vi "Get_Status.vi"(5 "Device Number":T1, 7 "Update":bool) -> (2 "Status":T4 {"OP Status" items=["INITIALIZING", "SELFTEST_IN_PROGRESS", "ERROR", "IMU_AUTOCAL_IN_PROGRESS", "NORMAL"]; "Calibration Status" items=["IMU_CAL_STATE_MASK"=3, "IMU_CAL_STATE_INPROGRESS"=0, "IMU_CAL_STATE_ACCUMULATE"=1, "IMU_CAL_STATE_COMPLETE"=2]})   [LabVIEW 2019]
doc: "This navX VI returns the current status of the navX."
uses:
  _TypeDefs/Flags/Z900_navX_Flags_OpStatusTypeDef.ctl
  _TypeDefs/Flags/Z900_navX_Flags_CalibrationStatusTypeDef.ctl
  _TypeDefs/FRIC_navX_DeviceNumbersTypeDef.ctl
  _TypeDefs/Z900_navX_DeviceRegisters.ctl
  _TypeDefs/Flags/Z900_navX_Flags_SelfTestStatusTypeDef.ctl
  _Util/Z900_navX_Util_LittleEndian_to_BigEndian.vi
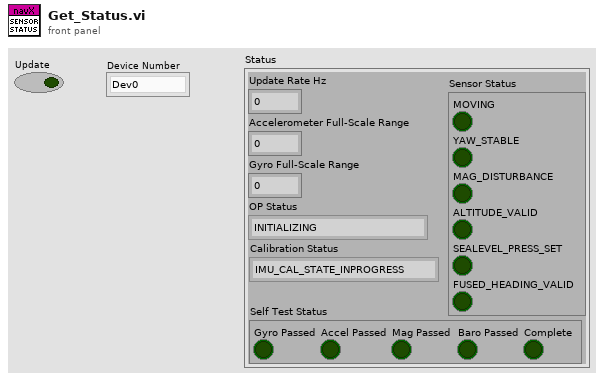
[diagram p1: front panel]
types:
  T1 = typedef "FRIC_navX_DeviceNumbersTypeDef.ctl" = enum16{"Dev0", "Dev1", "Dev2", "Dev3"}
  T2 = typedef "Z900_navX_Flags_OpStatusTypeDef.ctl" = u8
  T3 = typedef "Z900_navX_Flags_CalibrationStatusTypeDef.ctl" = u8
  T4 = cluster{"Update Rate Hz":u8, "Accelerometer Full-Scale Range":u8, "Gyro Full-Scale Range":u16, "OP Status":T2, "Calibration Status":T3, "Sensor Status":cluster{"MOVING":bool, "YAW_STABLE":bool, "MAG_DISTURBANCE":bool, "ALTITUDE_VALID":bool, "SEALEVEL_PRESS_SET":bool, "FUSED_HEADING_VALID":bool}, "Self Test Status":cluster{"Gyro Passed":bool, "Accel Passed":bool, "Mag Passed":bool, "Baro Passed":bool, "Complete":bool}}
  T5 = cluster{"MOVING":bool, "YAW_STABLE":bool, "MAG_DISTURBANCE":bool, "ALTITUDE_VALID":bool, "SEALEVEL_PRESS_SET":bool, "FUSED_HEADING_VALID":bool}
  T6 = cluster{"Gyro Passed":bool, "Accel Passed":bool, "Mag Passed":bool, "Baro Passed":bool, "Complete":bool}
  T7 = typedef "Z900_navX_Flags_SelfTestStatusTypeDef.ctl" = u8
  T8 = typedef "Z900_navX_DeviceRegisters.ctl" = u8
  T9 = cluster{"Update Rate Hz":u8, "Accelerometer Full-Scale Range":u8, "Gyro Full-Scale Range":u16, "OP Status":T2, "Calibration Status":T3, "Sensor Status":cluster{"MOVING":bool, "YAW_STABLE":bool, "MAG_DISTURBANCE":bool, "ALTITUDE_VALID":bool, "SEALEVEL_PRESS_SET":bool, "FUSED_HEADING_VALID":bool}, "Self Test Status":cluster{"Gyro Passed":bool, "Accel Passed":bool, "Mag Passed":bool, "Baro Passed":bool, "Complete":bool}}[]
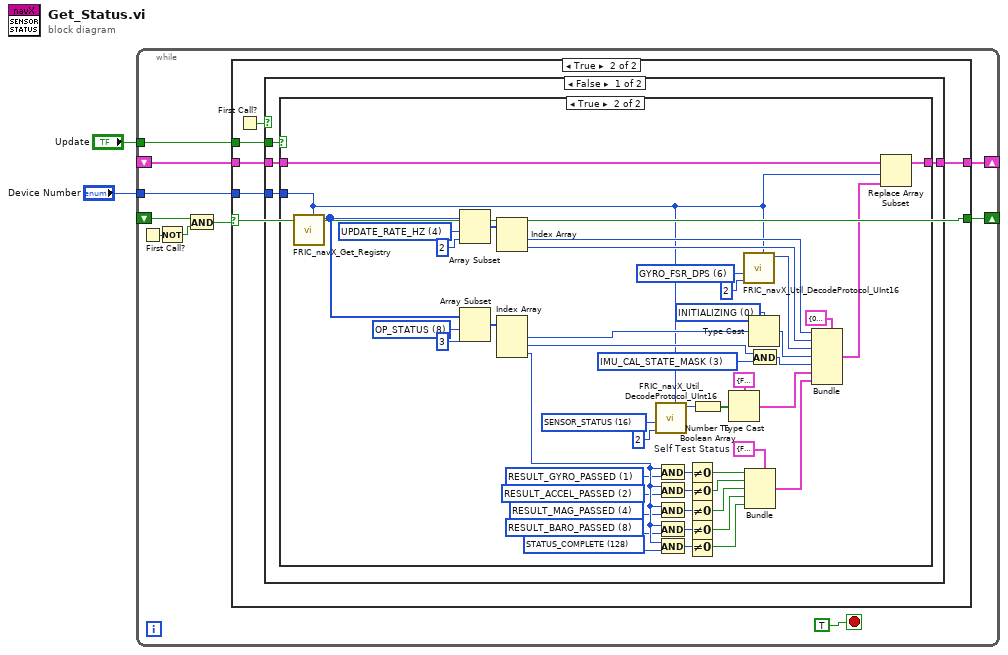
[diagram p0: block diagram]
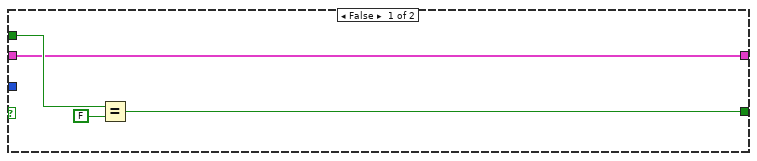
[diagram p2: hidden frame]
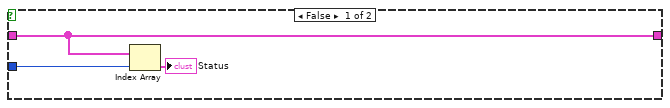
[diagram p3: hidden frame]
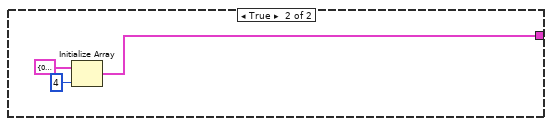
[diagram p4: hidden frame]
diagram:
  n1 = while {
    shift-right: [w12] -> _
    shift-left: _ -> [w9]
    tunnel: "Update" -> [w10]
    tunnel: "Device Number" -> [w8]
    shift-right: [w3] -> _
    shift-left: _ -> [w5]
    stop <- TRUE stop-if-true
    n2 = First Call?() -> (First Call?: T/F=w7:bool)
    n3 = Not(x=w7) -> (.not. x?=w6:bool)
    n4 = And(x=w5, y=w6) -> (x .and. y?=w4:bool)
    n5 = case shown="True" w4 {
      selector: w4 -> [_ w17]
      tunnel: [w13 w22] -> w12
      tunnel: w10 -> [w15 w21]
      tunnel: w9 -> [w13 w20]
      tunnel: w8 -> [_ w19]
      tunnel: [w14 w17] -> w3
      frame False {
        n6 = Equal?(x=w15, y=FALSE) -> (x = y?=w14:bool)
      }
      frame True {
        n7 = First Call?() -> (First Call?: T/F=w18:bool)
        n8 = case shown="False" w18 {
          tunnel: [w26 w77] -> w22
          tunnel: w21 -> [w25 _]
          tunnel: w20 -> [w24 _]
          tunnel: w19 -> [w23 _]
          frame False {
            n9 = case shown="True" w25 {
              tunnel: [w28 w32] -> w26
              tunnel: w24 -> [w28 w33]
              tunnel: w23 -> [w27 w30]
              frame False {
                n10 = Index Array(array=w28, index=w27) -> (element=→"Status":T4)
              }
              frame True {
                w34 = T6 {"Gyro Passed"=FALSE, "Accel Passed"=FALSE, "Mag Passed"=FALSE, "Baro Passed"=FALSE, "Complete"=FALSE}  # Self Test Status
                w41 = T7 128 items=["STATUS_COMPLETE"=128, "RESULT_GYRO_PASSED"=1, "RESULT_ACCEL_PASSED"=2, "RESULT_MAG_PASSED"=4, "RESULT_BARO_PASSED"=8] ("Self Test Status")
                w42 = T7 8 items=["STATUS_COMPLETE"=128, "RESULT_GYRO_PASSED"=1, "RESULT_ACCEL_PASSED"=2, "RESULT_MAG_PASSED"=4, "RESULT_BARO_PASSED"=8] ("Self Test Status")
                w45 = T7 4 items=["STATUS_COMPLETE"=128, "RESULT_GYRO_PASSED"=1, "RESULT_ACCEL_PASSED"=2, "RESULT_MAG_PASSED"=4, "RESULT_BARO_PASSED"=8] ("Self Test Status")
                w46 = T7 2 items=["STATUS_COMPLETE"=128, "RESULT_GYRO_PASSED"=1, "RESULT_ACCEL_PASSED"=2, "RESULT_MAG_PASSED"=4, "RESULT_BARO_PASSED"=8] ("Self Test Status")
                w49 = T7 1 items=["STATUS_COMPLETE"=128, "RESULT_GYRO_PASSED"=1, "RESULT_ACCEL_PASSED"=2, "RESULT_MAG_PASSED"=4, "RESULT_BARO_PASSED"=8] ("Self Test Status")
                w51 = T8 8 items=["WHOAMI"=0, "HW_REV"=1, "FW_VER_MAJOR"=2, "FW_VER_MINOR"=3, "UPDATE_RATE_HZ"=4, "ACCEL_FSR_G"=5, "GYRO_FSR_DPS"=6, "OP_STATUS"=8, "CAL_STATUS"=9, "SELFTEST_STATUS"=10, "CAPABILITY_FLAGS_L"=11, "CAPABILITY_FLAGS_H"=12, "SENSOR_STATUS"=16, "TIMESTAMP"=18, "YAW"=22, "ROLL"=24, "PITCH"=26, "HEADING"=28, "FUSED_HEADING"=30, "ALTITUDE_I"=32, "ALTITUDE_D"=34, "LINERA_ACC_X"=36, "LINERA_ACC_Y"=38, "LINERA_ACC_Z"=40, "QUAT_W"=42, "QUAT_X"=44, "QUAT_Y"=46, "QUAT_Z"=48, "MPU_TEMP_C"=50, "GYRO_X"=52, "GYRO_Y"=54, "GYRO_Z"=56, "ACC_X"=58, "ACC_Y"=60, "ACC_Z"=62, "MAG_X"=64, "MAG_Y"=66, "MAG_Z"=68, "PRESSURE_I"=70, "PRESSURE_D"=72, "PRESSURE_TEMP"=74, "YAW_OFFSET"=76, "QUAT_OFFSET_W"=78, "QUAT_OFFSET_X"=80, "QUAT_OFFSET_Y"=82, "QUAT_OFFSET_Z"=84, "INTEGRATION_CONTROL"=86, "VELOCITY_X"=88, "VELOCITY_Y"=92, "VELOCITY_Z"=96, "DISPLACMENT_X"=100, "DISPLACMENT_Y"=104, "DISPLACEMENT_Z"=108] ("Device Register")
                w53 = T8 4 items=["WHOAMI"=0, "HW_REV"=1, "FW_VER_MAJOR"=2, "FW_VER_MINOR"=3, "UPDATE_RATE_HZ"=4, "ACCEL_FSR_G"=5, "GYRO_FSR_DPS"=6, "OP_STATUS"=8, "CAL_STATUS"=9, "SELFTEST_STATUS"=10, "CAPABILITY_FLAGS_L"=11, "CAPABILITY_FLAGS_H"=12, "SENSOR_STATUS"=16, "TIMESTAMP"=18, "YAW"=22, "ROLL"=24, "PITCH"=26, "HEADING"=28, "FUSED_HEADING"=30, "ALTITUDE_I"=32, "ALTITUDE_D"=34, "LINERA_ACC_X"=36, "LINERA_ACC_Y"=38, "LINERA_ACC_Z"=40, "QUAT_W"=42, "QUAT_X"=44, "QUAT_Y"=46, "QUAT_Z"=48, "MPU_TEMP_C"=50, "GYRO_X"=52, "GYRO_Y"=54, "GYRO_Z"=56, "ACC_X"=58, "ACC_Y"=60, "ACC_Z"=62, "MAG_X"=64, "MAG_Y"=66, "MAG_Z"=68, "PRESSURE_I"=70, "PRESSURE_D"=72, "PRESSURE_TEMP"=74, "YAW_OFFSET"=76, "QUAT_OFFSET_W"=78, "QUAT_OFFSET_X"=80, "QUAT_OFFSET_Y"=82, "QUAT_OFFSET_Z"=84, "INTEGRATION_CONTROL"=86, "VELOCITY_X"=88, "VELOCITY_Y"=92, "VELOCITY_Z"=96, "DISPLACMENT_X"=100, "DISPLACMENT_Y"=104, "DISPLACEMENT_Z"=108] ("Device Register")
                w57 = T8 16 items=["WHOAMI"=0, "HW_REV"=1, "FW_VER_MAJOR"=2, "FW_VER_MINOR"=3, "UPDATE_RATE_HZ"=4, "ACCEL_FSR_G"=5, "GYRO_FSR_DPS"=6, "OP_STATUS"=8, "CAL_STATUS"=9, "SELFTEST_STATUS"=10, "CAPABILITY_FLAGS_L"=11, "CAPABILITY_FLAGS_H"=12, "SENSOR_STATUS"=16, "TIMESTAMP"=18, "YAW"=22, "ROLL"=24, "PITCH"=26, "HEADING"=28, "FUSED_HEADING"=30, "ALTITUDE_I"=32, "ALTITUDE_D"=34, "LINERA_ACC_X"=36, "LINERA_ACC_Y"=38, "LINERA_ACC_Z"=40, "QUAT_W"=42, "QUAT_X"=44, "QUAT_Y"=46, "QUAT_Z"=48, "MPU_TEMP_C"=50, "GYRO_X"=52, "GYRO_Y"=54, "GYRO_Z"=56, "ACC_X"=58, "ACC_Y"=60, "ACC_Z"=62, "MAG_X"=64, "MAG_Y"=66, "MAG_Z"=68, "PRESSURE_I"=70, "PRESSURE_D"=72, "PRESSURE_TEMP"=74, "YAW_OFFSET"=76, "QUAT_OFFSET_W"=78, "QUAT_OFFSET_X"=80, "QUAT_OFFSET_Y"=82, "QUAT_OFFSET_Z"=84, "INTEGRATION_CONTROL"=86, "VELOCITY_X"=88, "VELOCITY_Y"=92, "VELOCITY_Z"=96, "DISPLACMENT_X"=100, "DISPLACMENT_Y"=104, "DISPLACEMENT_Z"=108] ("Device Register")
                w60 = T8 6 items=["WHOAMI"=0, "HW_REV"=1, "FW_VER_MAJOR"=2, "FW_VER_MINOR"=3, "UPDATE_RATE_HZ"=4, "ACCEL_FSR_G"=5, "GYRO_FSR_DPS"=6, "OP_STATUS"=8, "CAL_STATUS"=9, "SELFTEST_STATUS"=10, "CAPABILITY_FLAGS_L"=11, "CAPABILITY_FLAGS_H"=12, "SENSOR_STATUS"=16, "TIMESTAMP"=18, "YAW"=22, "ROLL"=24, "PITCH"=26, "HEADING"=28, "FUSED_HEADING"=30, "ALTITUDE_I"=32, "ALTITUDE_D"=34, "LINERA_ACC_X"=36, "LINERA_ACC_Y"=38, "LINERA_ACC_Z"=40, "QUAT_W"=42, "QUAT_X"=44, "QUAT_Y"=46, "QUAT_Z"=48, "MPU_TEMP_C"=50, "GYRO_X"=52, "GYRO_Y"=54, "GYRO_Z"=56, "ACC_X"=58, "ACC_Y"=60, "ACC_Z"=62, "MAG_X"=64, "MAG_Y"=66, "MAG_Z"=68, "PRESSURE_I"=70, "PRESSURE_D"=72, "PRESSURE_TEMP"=74, "YAW_OFFSET"=76, "QUAT_OFFSET_W"=78, "QUAT_OFFSET_X"=80, "QUAT_OFFSET_Y"=82, "QUAT_OFFSET_Z"=84, "INTEGRATION_CONTROL"=86, "VELOCITY_X"=88, "VELOCITY_Y"=92, "VELOCITY_Z"=96, "DISPLACMENT_X"=100, "DISPLACMENT_Y"=104, "DISPLACEMENT_Z"=108] ("Device Register")
                w72 = T3 3 items=["IMU_CAL_STATE_MASK"=3, "IMU_CAL_STATE_INPROGRESS"=0, "IMU_CAL_STATE_ACCUMULATE"=1, "IMU_CAL_STATE_COMPLETE"=2] ("CalibrationStatus")
                w74 = T2 0 items=["INITIALIZING", "SELFTEST_IN_PROGRESS", "ERROR", "IMU_AUTOCAL_IN_PROGRESS", "NORMAL"] ("OP Status")
                n11 = call "FRIC_navX_Get_Registry.vi"("Device Number"=w30) -> ("Registry (out)"=w50:u8[])  [unwired: 9 in, 1 out]
                n12 = Array Subset(array=w50, index=w53, length=2) -> (w66:u8[])
                n13 = Array Subset(array=w50, index=w51, length=3) -> (w76:u8[])
                n14 = Index Array(array=w66) -> (element #1=w64:u8, element #2=w65:u8)  [unwired: 2 in]
                n15 = Index Array(array=w76) -> (element #1=w75:u8, element #2=w73:u8, element #3=w63:u8)  [unwired: 3 in]
                n16 = call "FRIC_navX_Util_DecodeProtocol_UInt16.vi"("Device Number"=w30, "length"=2, "Device Register"=w57) -> ("Value"=w55:u16)  [unwired: 8 in]
                n17 = And(x=w63, y=w49) -> (x .and. y?=w48:T7)
                n18 = And(x=w63, y=w46) -> (x .and. y?=w47:T7)
                n19 = And(x=w63, y=w45) -> (x .and. y?=w44:T7)
                n20 = And(x=w63, y=w42) -> (x .and. y?=w43:T7)
                n21 = And(x=w63, y=w41) -> (x .and. y?=w40:T7)
                n22 = Not Equal To 0?(x=w48) -> (x != 0?=w39:bool)
                n23 = Not Equal To 0?(x=w47) -> (x != 0?=w38:bool)
                n24 = Not Equal To 0?(x=w44) -> (x != 0?=w37:bool)
                n25 = Not Equal To 0?(x=w43) -> (x != 0?=w36:bool)
                n26 = Not Equal To 0?(x=w40) -> (x != 0?=w35:bool)
                n27 = Number To Boolean Array(number=w55) -> (Boolean array=w68:bool[])
                n28 = Type Cast(type=T5 {"MOVING"=FALSE, "YAW_STABLE"=FALSE, "MAG_DISTURBANCE"=FALSE, "ALTITUDE_VALID"=FALSE, "SEALEVEL_PRESS_SET"=FALSE, "FUSED_HEADING_VALID"=FALSE} ("NAVX_SENSOR_STATUS"), x=w68) -> (*(type *) &x=w62:T5)
                n29 = call "FRIC_navX_Util_DecodeProtocol_UInt16.vi"("Device Number"=w30, "length"=2, "Device Register"=w60) -> ("Value"=w58:u16)  [unwired: 8 in]
                n30 = Bundle(cluster=w34, "Gyro Passed"=w39, "Accel Passed"=w38, "Mag Passed"=w37, "Baro Passed"=w36, "Complete"=w35) -> (w61:T6)
                n31 = Type Cast(type=w74, x=w75) -> (*(type *) &x=w70:T2)
                n32 = And(x=w73, y=w72) -> (x .and. y?=w69:T3)
                n33 = Bundle(cluster=T4 {"Update Rate Hz"=0, "Accelerometer Full-Scale Range"=0, "Gyro Full-Scale Range"=0, "OP Status"=0, "Calibration Status"=3, "Sensor Status"={"MOVING"=FALSE, "YAW_STABLE"=FALSE, "MAG_DISTURBANCE"=FALSE, "ALTITUDE_VALID"=FALSE, "SEALEVEL_PRESS_SET"=FALSE, "FUSED_HEADING_VALID"=FALSE}, "Self Test Status"={"Gyro Passed"=FALSE, "Accel Passed"=FALSE, "Mag Passed"=FALSE, "Baro Passed"=FALSE, "Complete"=FALSE}}, "Update Rate Hz"=w64, "Accelerometer Full-Scale Range"=w65, "Gyro Full-Scale Range"=w58, "OP Status"=w70, "Calibration Status"=w69, "Sensor Status"=w62, "Self Test Status"=w61) -> (w31:T4)
                n34 = Replace Array Subset(array=w33, new element=w31, index=w30) -> (w32:T9)
              }
            }
          }
          frame True {
            n35 = Initialize Array(T4 {"Update Rate Hz"=0, "Accelerometer Full-Scale Range"=0, "Gyro Full-Scale Range"=0, "OP Status"=0, "Calibration Status"=0, "Sensor Status"={"MOVING"=FALSE, "YAW_STABLE"=FALSE, "MAG_DISTURBANCE"=FALSE, "ALTITUDE_VALID"=FALSE, "SEALEVEL_PRESS_SET"=FALSE, "FUSED_HEADING_VALID"=FALSE}, "Self Test Status"={"Gyro Passed"=FALSE, "Accel Passed"=FALSE, "Mag Passed"=FALSE, "Baro Passed"=FALSE, "Complete"=FALSE}}, 4 ("dimension size")) -> (w77:T9)
          }
        }
      }
    }
  }
